vi "PMBus Read Byte Ext.vi"(4 "PEC":u8, 5 "CommandCode":u8, 6 "CommandCodeExt":u8, 7 "SlaveAddr":u8, 9 "PMBusIndex":i32, 10 "DevIndex":i32, 11 "DevType":i32) -> (2 "function return":i32, 3 "pData":u8)   [LabVIEW 2010, in "ControlPMBus.lvlib"]
doc: "int WINAPI PMBus_ReadByteExt(int DevType,int DevIndex,int PMBusIndex,unsigned char SlaveAddr,unsigned char CommandCodeExt,unsigned char CommandCode, unsigned char *pData,unsigned char PEC);"
uses:
  ControlPMBus.lvlib
  ControlPMBus/Ginkgo_Driver.dll
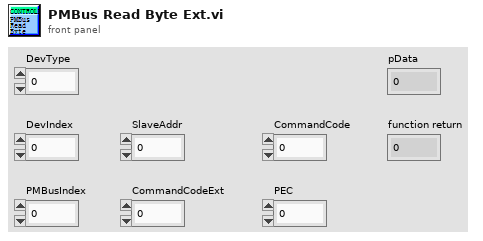
[diagram p1: front panel]
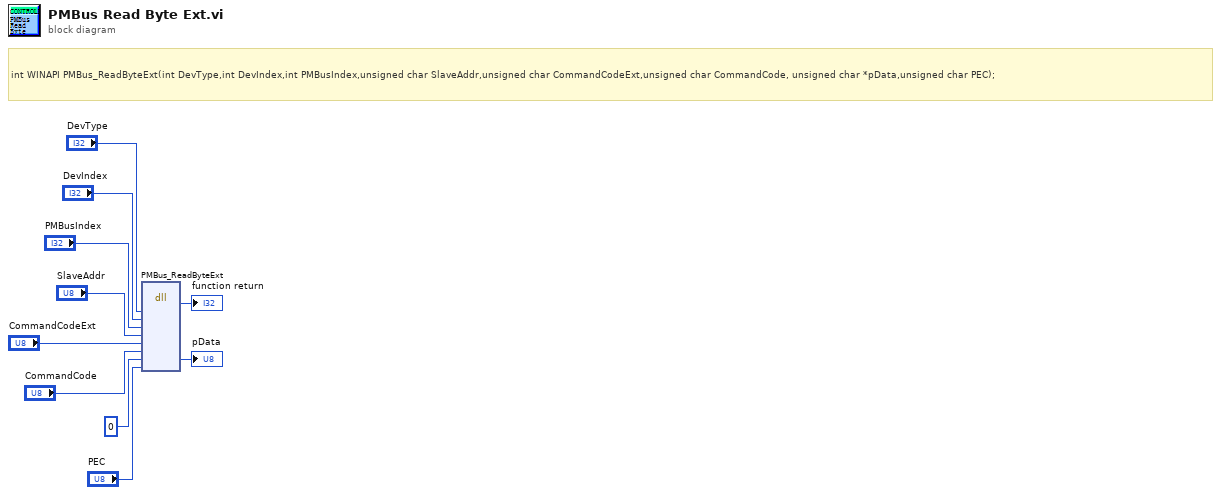
[diagram p0: block diagram]
diagram:
  # "int WINAPI PMBus_ReadByteExt(int DevType,int DevIndex,int PMBusIndex,unsigned char SlaveAddr,unsigned char CommandCodeExt,unsigned char CommandCode, unsigned char *pData,unsigned char PEC);"
  n1 = dll-call lib="E:/Project/vt_ginkgo/truck/Ginkgo Driver/vs2010/Ginkgo_USB-I2C&SPI&CAN_API_v2.0.3.3/lib/labview_32bit/ControlPMBus/Ginkgo_Driver.*" fn="PMBus_ReadByteExt"("DevType"="DevType", "DevIndex"="DevIndex", "PMBusIndex"="PMBusIndex", "SlaveAddr"="SlaveAddr", "CommandCodeExt"="CommandCodeExt", "CommandCode"="CommandCode", "pData"=u8 0, "PEC"="PEC") -> (→"function return":i32, "pData"=→"pData":u8)  [unwired: 10 in, 2 out]
